vi "cfg combine v2 and v3.vi"(8 "error in":errorcluster, 10 "Log Actions":T1(array[cluster]), 11 "Engine Configuration In":T3(array[cluster])) -> (0 "error out":errorcluster, 3 "Engine Configuration Out":T4[](array[typedef]))   [LabVIEW 2013, in "Standard Engine Configuration.lvclass"]
uses:
  Standard Engine Configuration.lvclass
  Module Specific Configuration.ctl
  Module Decimation.ctl
  Runtime/error responses.ctl
  error options.ctl
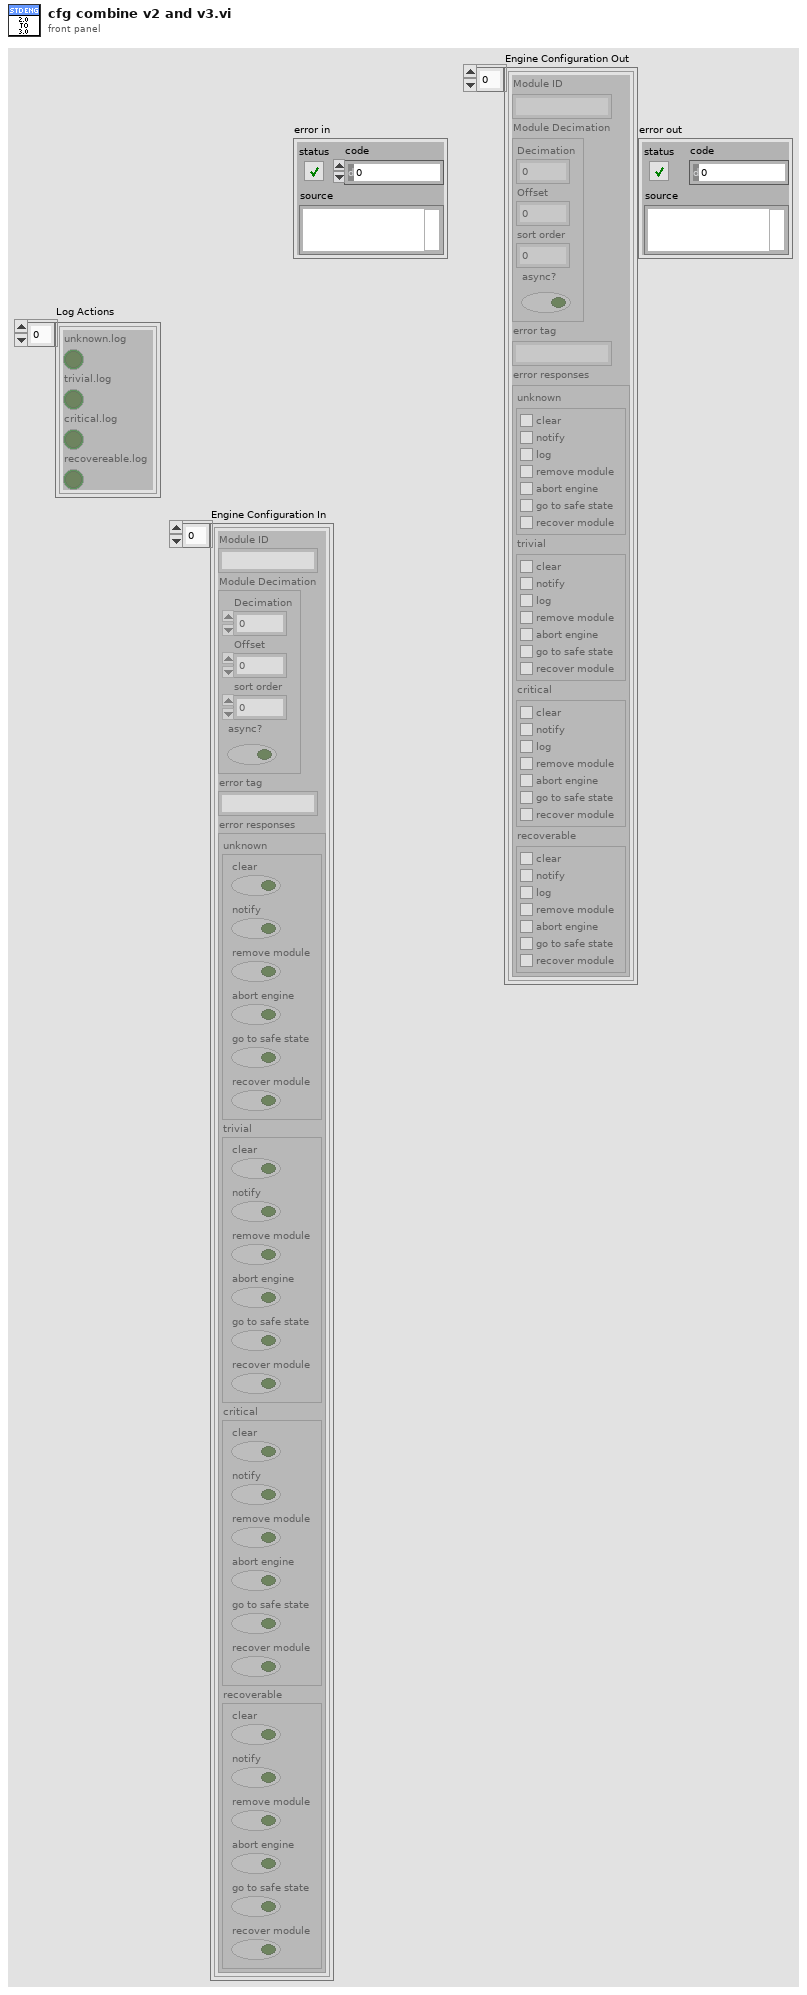
[diagram p1: front panel]
types:
  T1 = cluster{"unknown.log":bool, "trivial.log":bool, "critical.log":bool, "recovereable.log":bool}[]
  T2 = typedef "Standard Engine Configuration.lvclass/Module Decimation.ctl" = cluster{"Decimation":u16, "Offset":u16, "sort order":i32, "async?":bool}
  T3 = cluster{"Module ID":string, "Module Decimation":T2, "error tag":string, "error responses":cluster{"unknown":cluster{"clear":bool, "notify":bool, "remove module":bool, "abort engine":bool, "go to safe state":bool, "recover module":bool}, "trivial":cluster{"clear":bool, "notify":bool, "remove module":bool, "abort engine":bool, "go to safe state":bool, "recover module":bool}, "critical":cluster{"clear":bool, "notify":bool, "remove module":bool, "abort engine":bool, "go to safe state":bool, "recover module":bool}, "recoverable":cluster{"clear":bool, "notify":bool, "remove module":bool, "abort engine":bool, "go to safe state":bool, "recover module":bool}}}[]
  T4 = typedef "Standard Engine Configuration.lvclass/Module Specific Configuration.ctl" = cluster{"Module ID":string, "Module Decimation":T2, "error tag":string, "error responses":T5}
  T5 = typedef "Standard Engine Configuration.lvclass/error responses.ctl" = cluster{"unknown":T6, "trivial":T6, "critical":T6, "recoverable":T6}
  T6 = typedef "Standard Engine Configuration.lvclass/error options.ctl" = cluster{"clear":bool, "notify":bool, "log":bool, "remove module":bool, "abort engine":bool, "go to safe state":bool, "recover module":bool}
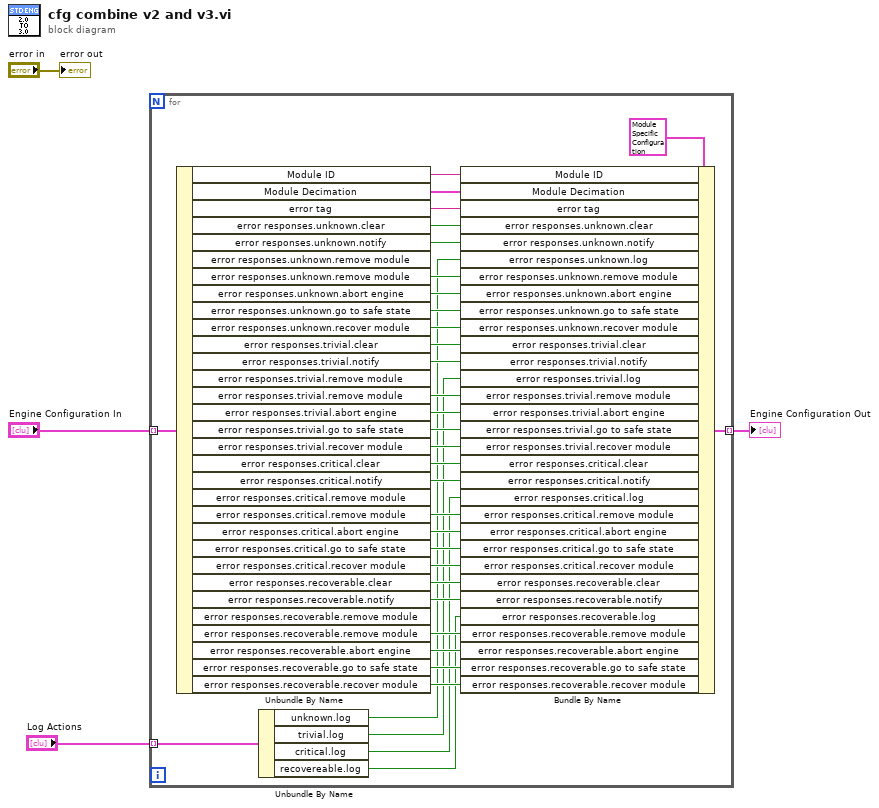
[diagram p0: block diagram]
diagram:
  n1 = for {
    tunnel: "Engine Configuration In" -> [w39] mode=indexing
    tunnel: [w37] -> w2 mode=indexing
    tunnel: "Log Actions" -> [w9] mode=indexing
    n2 = Unbundle By Name(w39) -> ("Module ID"=w36:string, "Module Decimation"=w35:T2, "error tag"=w34:string, "error responses.unknown.clear"=w33:bool, "error responses.unknown.notify"=w32:bool, "error responses.unknown.remove module"=w28:bool, "error responses.unknown.abort engine"=w29:bool, "error responses.unknown.go to safe state"=w31:bool, "error responses.unknown.recover module"=w30:bool, "error responses.trivial.clear"=w27:bool, "error responses.trivial.notify"=w26:bool, "error responses.trivial.remove module"=w25:bool, "error responses.trivial.abort engine"=w24:bool, "error responses.trivial.go to safe state"=w23:bool, "error responses.trivial.recover module"=w22:bool, "error responses.critical.clear"=w21:bool, "error responses.critical.notify"=w20:bool, "error responses.critical.remove module"=w19:bool, "error responses.critical.abort engine"=w18:bool, "error responses.critical.go to safe state"=w17:bool, "error responses.critical.recover module"=w16:bool, "error responses.recoverable.clear"=w15:bool, "error responses.recoverable.notify"=w14:bool, "error responses.recoverable.remove module"=w13:bool, "error responses.recoverable.abort engine"=w12:bool, "error responses.recoverable.go to safe state"=w11:bool, "error responses.recoverable.recover module"=w10:bool)  [unwired: 4 out]
    n3 = Unbundle By Name(w9) -> ("unknown.log"=w8:bool, "trivial.log"=w7:bool, "critical.log"=w6:bool, "recovereable.log"=w5:bool)
    n4 = Bundle By Name(cluster=T4 {"Module ID"="", "Module Decimation"={"Decimation"=0, "Offset"=0, "sort order"=0, "async?"=FALSE}, "error tag"="", "error responses"={"unknown"={"clear"=FALSE, "notify"=FALSE, "log"=FALSE, "remove module"=FALSE, "abort engine"=FALSE, "go to safe state"=FALSE, "recover module"=FALSE}, "trivial"={"clear"=FALSE, "notify"=FALSE, "log"=FALSE, "remove module"=FALSE, "abort engine"=FALSE, "go to safe state"=FALSE, "recover module"=FALSE}, "critical"={"clear"=FALSE, "notify"=FALSE, "log"=FALSE, "remove module"=FALSE, "abort engine"=FALSE, "go to safe state"=FALSE, "recover module"=FALSE}, "recoverable"={"clear"=FALSE, "notify"=FALSE, "log"=FALSE, "remove module"=FALSE, "abort engine"=FALSE, "go to safe state"=FALSE, "recover module"=FALSE}}} ("Module Specific Configuration"), "Module ID"=w36, "Module Decimation"=w35, "error tag"=w34, "error responses.unknown.clear"=w33, "error responses.unknown.notify"=w32, "error responses.unknown.log"=w8, "error responses.unknown.remove module"=w28, "error responses.unknown.abort engine"=w29, "error responses.unknown.go to safe state"=w31, "error responses.unknown.recover module"=w30, "error responses.trivial.clear"=w27, "error responses.trivial.notify"=w26, "error responses.trivial.log"=w7, "error responses.trivial.remove module"=w25, "error responses.trivial.abort engine"=w24, "error responses.trivial.go to safe state"=w23, "error responses.trivial.recover module"=w22, "error responses.critical.clear"=w21, "error responses.critical.notify"=w20, "error responses.critical.log"=w6, "error responses.critical.remove module"=w19, "error responses.critical.abort engine"=w18, "error responses.critical.go to safe state"=w17, "error responses.critical.recover module"=w16, "error responses.recoverable.clear"=w15, "error responses.recoverable.notify"=w14, "error responses.recoverable.log"=w5, "error responses.recoverable.remove module"=w13, "error responses.recoverable.abort engine"=w12, "error responses.recoverable.go to safe state"=w11, "error responses.recoverable.recover module"=w10) -> (w37:T4)
  }
  "Engine Configuration Out" <- w2
  "error out" <- "error in"
